vi "Z Aux Set Trace File.vi"(8 "error in (no error)":errorcluster caption="错误输入（无错误）", 10 "pFilePathName":string, 11 "bifTofile":i32) -> (0 "error out":errorcluster caption="错误输出", 3 "function return":i32)   [LabVIEW 2015, in "zauxdll.lvlib"]
doc: "int32 __stdcall ZAux_SetTraceFile(int bifTofile, const char *pFilePathName);"
uses:
  zauxdll.lvlib
  zauxdll.dll
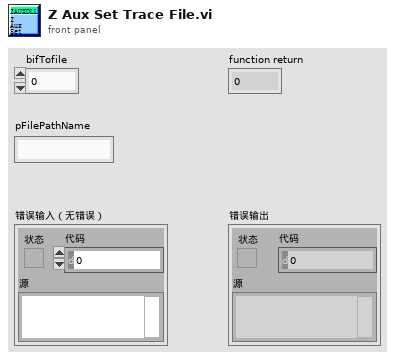
[diagram p1: front panel]
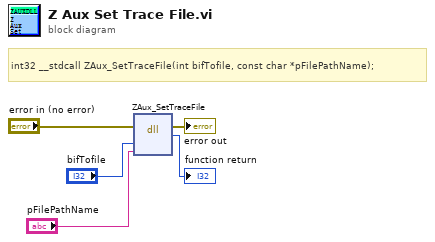
[diagram p0: block diagram]
diagram:
  # "int32 __stdcall ZAux_SetTraceFile(int bifTofile, const char *pFilePathName);"
  n1 = dll-call lib="C:/Users/VIC/Desktop/GOGORO_Oringnal - Panasonic/system/LLB/zmotion/zaux/zauxdll.*" fn="ZAux_SetTraceFile"(error in="error in (no error)", "bifTofile"="bifTofile", "pFilePathName"="pFilePathName") -> (error out=→"error out":errorcluster, →"function return":i32)  [unwired: 4 in, 1 out]
